vi "close_app_ref.vi"(11 "app_ref":u32) -> ()   [LabVIEW 2024]
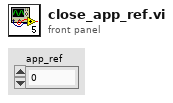
[diagram p1: front panel]
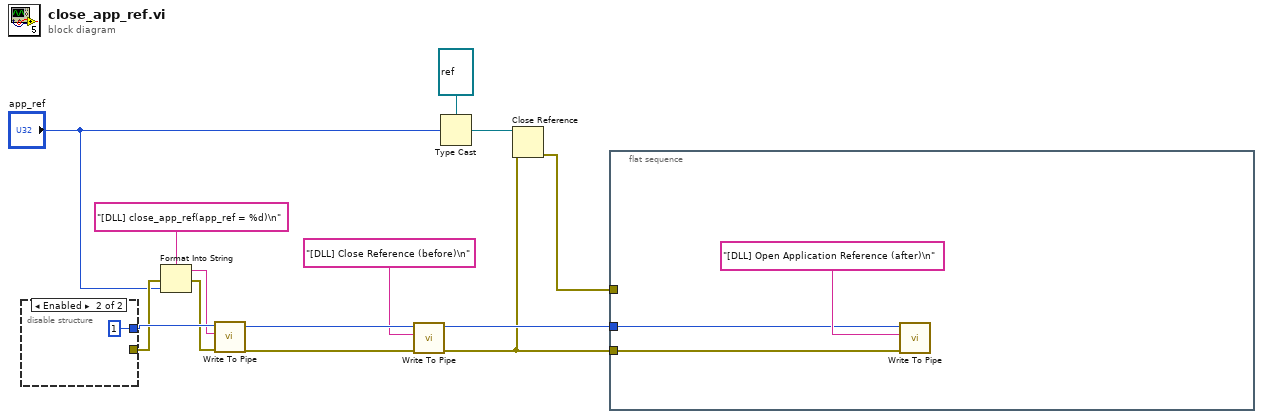
[diagram p0: block diagram]
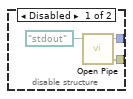
[diagram p2: hidden frame]
diagram:
  n1 = disable-structure shown="Enabled" {
    disable-tunnel: [w16 1 ("file descriptor")] -> w12
    disable-tunnel: [w15 _] -> w10
    frame Disabled {
      n2 = call <vilib>:"Open Pipe.vi"("path to named pipe"=path "stdout") -> ("error out"=w15:errorcluster, "file descriptor"=w16:i32)  [unwired: 3 in]
    }
    frame Enabled {
    }
  }
  n3 = Format Into String(format string="[DLL] close_app_ref(app_ref = %d)\n", error in=w10, "app_ref") -> (resulting string=w8:string, error out=w9:errorcluster)  [unwired: 1 in]
  n4 = call <vilib>:"Write To Pipe.vi"("error in (no error)"=w9, "data"=w8, "file descriptor"=w12) -> ("error out"=w5:errorcluster, "file descriptor"=w7:i32)  [unwired: 2 in, 1 out]
  n5 = call <vilib>:"Write To Pipe.vi"("error in (no error)"=w5, "data"="[DLL] Close Reference (before)\n" ("format string"), "file descriptor"=w7) -> ("error out"=w2:errorcluster, "file descriptor"=w4:i32)  [unwired: 2 in, 1 out]
  n6 = Type Cast(type=refnum<vi> refnum ("application reference"), x="app_ref") -> (*(type *) &x=w14:refnum<vi>)
  n7 = Close Reference(reference=w14, error in (no error)=w2) -> (error out=w3:errorcluster)
  n8 = flat-sequence {
    tunnel: w4 -> [w20]
    tunnel: w3 -> [_]
    tunnel: w2 -> [w19]
    frame #0 {
      n9 = call <vilib>:"Write To Pipe.vi"("error in (no error)"=w19, "data"="[DLL] Open Application Reference (after)\n" ("format string"), "file descriptor"=w20) -> ()  [unwired: 2 in, 3 out]
    }
  }
